vi "SetWaveColor.vi"() -> ()   [LabVIEW 2012]
uses:
  <vilib>/measure/NI_MABase.lvlib
panel:
  in  "颜色盒 8":u32(colorbox)
  in  "颜色盒 7":u32(colorbox)
  in  "颜色盒 6":u32(colorbox)
  in  "颜色盒 5":u32(colorbox)
  out "颜色盒 4":u32(colorbox)
  out "颜色盒 3":u32(colorbox)
  out "颜色盒 2":u32(colorbox)
  out "颜色盒":u32(colorbox)
  out "波形图":waveform(dbl)[](graph)
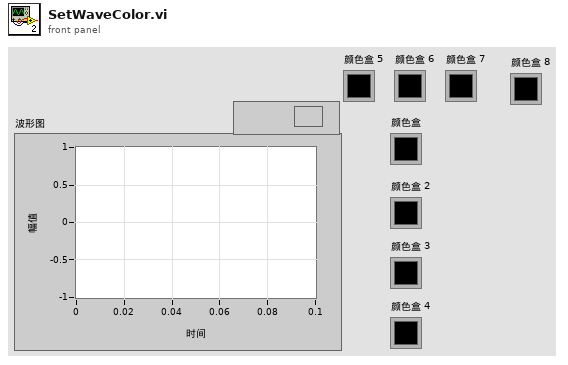
[diagram p1: front panel]
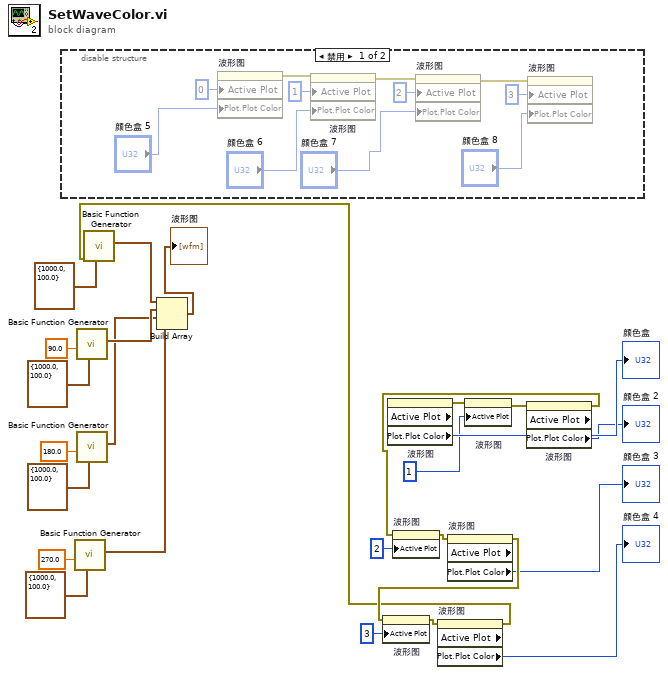
[diagram p0: block diagram]
diagram:
  n1 = disable-structure shown="禁用" {
    frame Disabled {
      n2 = property on="波形图" class="WFGraph (严格)"("Active Plot"=u32 0 ("活动曲线"), "Plot.Plot Color"="颜色盒 5") -> (error out=w37:errorcluster)  [unwired: 2 in, 1 out]
      n3 = property on="波形图" class="WFGraph (严格)"(error in=w37, "Active Plot"=u32 1 ("活动曲线"), "Plot.Plot Color"="颜色盒 6") -> (error out=w35:errorcluster)  [unwired: 1 in, 1 out]
      n4 = property on="波形图" class="WFGraph (严格)"(error in=w35, "Active Plot"=u32 2 ("活动曲线"), "Plot.Plot Color"="颜色盒 7") -> (error out=w36:errorcluster)  [unwired: 1 in, 1 out]
      n5 = property on="波形图" class="WFGraph (严格)"(error in=w36, "Active Plot"=u32 3 ("活动曲线"), "Plot.Plot Color"="颜色盒 8") -> ()  [unwired: 1 in, 2 out]
    }
    frame Enabled {
    }
  }
  n6 = call <vilib>:"Basic Function Generator.vi"("sampling info"=cluster{"Fs":dbl, "#s":dbl} {"Fs"=1000.0, "#s"=100.0}, "phase"=270.0) -> ("signal out"=w2:waveform(dbl))  [unwired: 7 in, 2 out]
  n7 = call <vilib>:"Basic Function Generator.vi"("sampling info"=cluster{"Fs":dbl, "#s":dbl} {"Fs"=1000.0, "#s"=100.0}, "phase"=90.0) -> ("signal out"=w18:waveform(dbl))  [unwired: 7 in, 2 out]
  n8 = call <vilib>:"Basic Function Generator.vi"("sampling info"=cluster{"Fs":dbl, "#s":dbl} {"Fs"=1000.0, "#s"=100.0}, "phase"=180.0) -> ("signal out"=w17:waveform(dbl))  [unwired: 7 in, 2 out]
  n9 = property on="波形图" class="WFGraph (严格)" props=["Active Plot", "Plot", "Plot Color"]() -> (error out=w13:errorcluster, "Plot.Plot Color"=→"颜色盒":u32)  [unwired: 2 in, 2 out]
  n10 = property on="波形图" class="WFGraph (严格)"(error in=w13, "Active Plot"=u32 1 ("活动曲线")) -> (error out=w12:errorcluster)  [unwired: 1 in, 1 out]
  n11 = property on="波形图" class="WFGraph (严格)" props=["Active Plot", "Plot", "Plot Color"](error in=w12) -> (error out=w7:errorcluster, "Plot.Plot Color"=→"颜色盒 2":u32)  [unwired: 1 in, 2 out]
  n12 = property on="波形图" class="WFGraph (严格)"(error in=w7, "Active Plot"=u32 2 ("活动曲线")) -> (error out=w10:errorcluster)  [unwired: 1 in, 1 out]
  n13 = property on="波形图" class="WFGraph (严格)" props=["Active Plot", "Plot", "Plot Color"](error in=w10) -> (error out=w6:errorcluster, "Plot.Plot Color"=→"颜色盒 3":u32)  [unwired: 1 in, 2 out]
  n14 = property on="波形图" class="WFGraph (严格)"(error in=w6, "Active Plot"=u32 3 ("活动曲线")) -> (error out=w5:errorcluster)  [unwired: 1 in, 1 out]
  n15 = property on="波形图" class="WFGraph (严格)" props=["Active Plot", "Plot", "Plot Color"](error in=w5) -> (error out=w1:errorcluster, "Plot.Plot Color"=→"颜色盒 4":u32)  [unwired: 1 in, 2 out]
  n16 = call <vilib>:"Basic Function Generator.vi"("sampling info"=cluster{"Fs":dbl, "#s":dbl} {"Fs"=1000.0, "#s"=100.0}, "error in (no error)"=w1) -> ("signal out"=w19:waveform(dbl))  [unwired: 7 in, 2 out]
  n17 = Build Array(w19, w18, w17, w2) -> (→"波形图":waveform(dbl)[])
